vi "Launch Debuggers.vi"(8 "error in (no error)":errorcluster, 11 "Volatus Core in":refnum<class "Volatus Core.lvclass">) -> (0 "error out":errorcluster, 3 "Volatus Core out":refnum<class "Volatus Core.lvclass">)   [LabVIEW 2020, in "Volatus.lvlib" / "Volatus Core.lvclass"]
uses:
  Volatus Core.lvclass
  C:/dev/lv20CE/relink/lv-volatus/Volatus/Module/Module.lvclass
  Debug Launcher/Debug Launcher.lvclass
  Volatus Core.lvclass/Volatus Core.ctl
  C:/dev/lv20CE/relink/lv-volatus/Volatus/Volatus Core/Volatus Core.lvclass
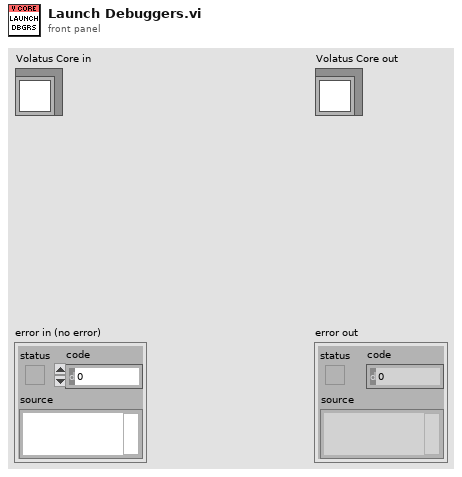
[diagram p1: front panel]
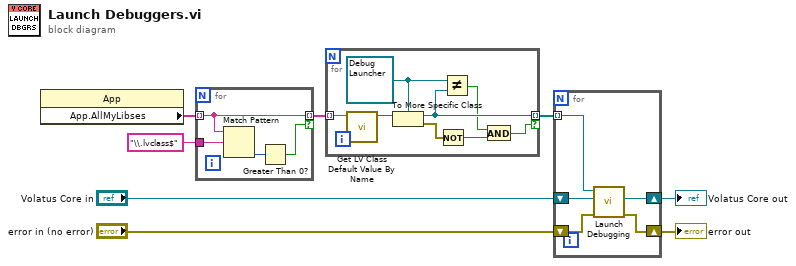
[diagram p0: block diagram]
diagram:
  n1 = property class="App"() -> ("App.AllMyLibses"=w8:string[])  [unwired: 2 in, 2 out]
  n2 = for {
    tunnel: w8 -> [w12] mode=indexing
    tunnel: [w12] -> w6 mode=indexing if=w9
    tunnel: "\\.lvclass$" -> [w11]
    n3 = Match Pattern(string=w12, regular expression=w11) -> (offset past match=w10:i32)  [unwired: 1 in, 3 out]
    n4 = Greater Than 0?(x=w10) -> (x > 0?=w9:bool)
  }
  n5 = for {
    tunnel: w6 -> [w20] mode=indexing
    tunnel: [w15] -> w5 mode=indexing if=w14
    w16 = refnum<class "Debug Launcher.lvclass"> refnum ("Volatus:Debug Launcher.lvclass")
    n6 = call <vilib>:"Get LV Class Default Value By Name.vi"("class name"=w20) -> ("object"=w19:refnum<class>)  [unwired: 9 in, 1 out]
    n7 = To More Specific Class(target class=w16, reference=w19) -> (specific class reference=w15:refnum<class "Debug Launcher.lvclass">, error out=w18:errorcluster)  [unwired: 1 in]
    n8 = Not(x=w18) -> (.not. x?=w17:bool)
    n9 = Not Equal?(x=w16, y=w15) -> (x != y?=w13:bool)
    n10 = And(x=w13, y=w17) -> (x .and. y?=w14:bool)
  }
  n11 = for {
    tunnel: w5 -> [w23] mode=indexing
    shift-right: [w24] -> w1
    shift-left: "Volatus Core in" -> [w25]
    shift-right: [w21] -> w2
    shift-left: "error in (no error)" -> [w22]
    n12 = call "Launch Debugging.vi"("error in (no error)"=w22, "Parent In"=w25, "Debug Launcher in"=w23) -> ("error out"=w21:errorcluster, "Parent"=w24:refnum<class "Volatus Core.lvclass">)  [unwired: 7 in]
  }
  "error out" <- w2
  "Volatus Core out" <- w1
